vi "WS1021 GUI.vi"() -> ()   [LabVIEW 2020, in "WS1021.lvclass"]
uses:
  WS1021.lvclass
  C:/Sandbox/Git_Sandbox/WiSpry Test Framework source code (LV20)/WiSpry Test Framework/Devices/PIC-device/PIC-Device.lvclass
  C:/Sandbox/Git_Sandbox/WiSpry Test Framework source code (LV20)/WiSpry Test Framework/Devices/Toggle 8/Toggle 8.lvclass
  C:/Sandbox/Git_Sandbox/WiSpry Test Framework source code (LV20)/WiSpry Test Framework/Devices/Device.lvclass
  Controls/Register to Write.ctl
  PIC-device/PIC-Device.lvclass/PIC-Device.ctl
  Private/Get register for reading - array.vi
  PIC-device/PIC-Device.lvclass
  Toggle 8.lvclass
panel:
  in  "Init part":bool
  out "Y":i32
  out "X":i32
  in  "All reg 2 & 3":bool
  in  "Beam control mode":enum32{"OTP calibration", "Direct control"}(radio)
  in  "All reg3":bool
  in  "All reg2":bool
  in  "Reg3 beams":string="TB1 \n1/4pF\n\nTB2 \n1/4pF\n\nTB3\n1/4pF\n\nTB4\n1/4pF\n\nTB5\n1/4pF\n\nFB3\n1/8pF\n\nFB1 \n1/32pF"
  in  "Reg2 beams":string="TB6 \n1/4pF\n\nTB7 \n1/4pF\n\nTB8 \n1/4pF\n\nTB9 \n1/4pF\n\nTB10 \n1/4pF\n\nTB11 \n1/4pF\n\nFB2 \n1/16pF"
  in  "Reg3":bool[](array[boolean])=[FALSE, FALSE, FALSE, FALSE, FALSE, FALSE, FALSE]
  in  "Reg2":bool[](array[boolean])=[FALSE, FALSE, FALSE, FALSE, FALSE, FALSE, FALSE]
  in  "Stop Button":bool
  out "Boolean":bool
  out "Cycle":i32=1
  in  "Cycles":i32=1
  in  "USID":bool=TRUE
  out "Connected":bool
  out "SN#":string
  out "Product ID":string
  out "Manufacturer ID":string
  in  "Read info [F5]":bool
  in  "Close connection":bool
  in  "Toggle beams":bool
  in  "OTP values to read":string="0:127/1"
  in  "Read OTP":bool
  in  "Toggle Cmin/Cmax":bool
  in  "Init":bool
  out "Error Out":errorcluster
  in  "Error In":errorcluster
  in  "Write":bool
  in  "Exit":bool
  in  "Read":bool
  in  "Read reg":string="076000"
  in  "Write reg":string="074220"
  out "Cmd Send out":string
  in  "VISA resource name":refnum<visa-resource-name>
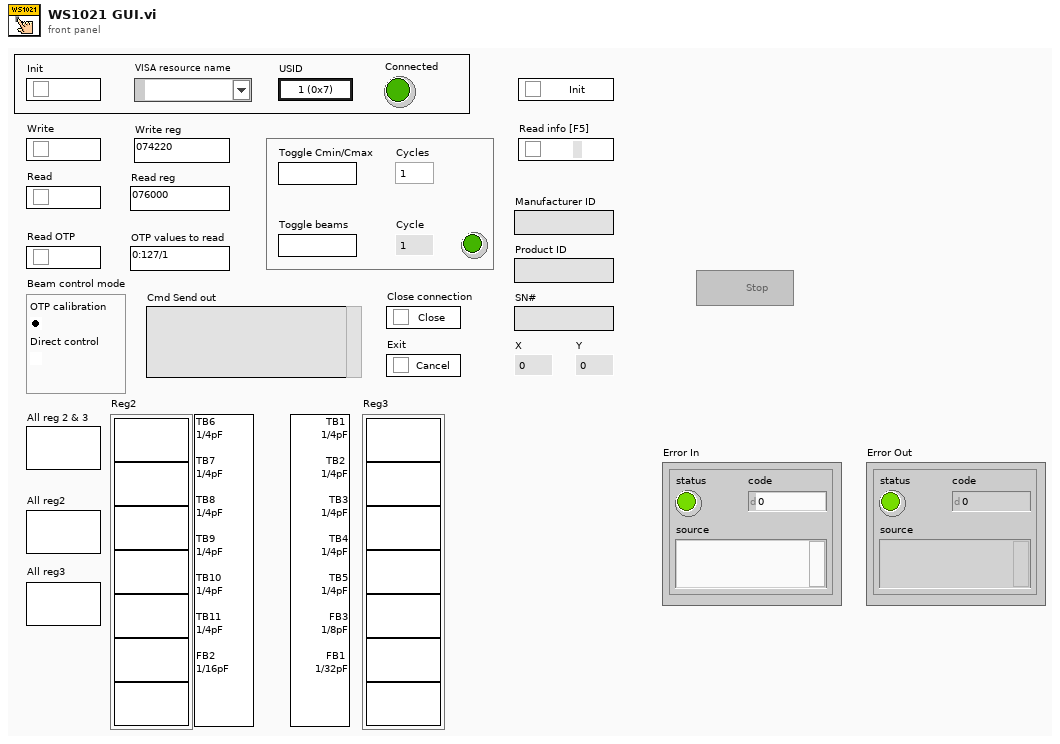
[diagram p1: front panel]
types:
  T1 = typedef "PIC-Device.lvclass/Register to Write.ctl" = cluster{"Register":u32, "Value":u32, "Dev Address":u32, "Physical Adress":u32}
  T2 = enum8{"Enabled", "Disabled", "Disabled and Grayed Out"}
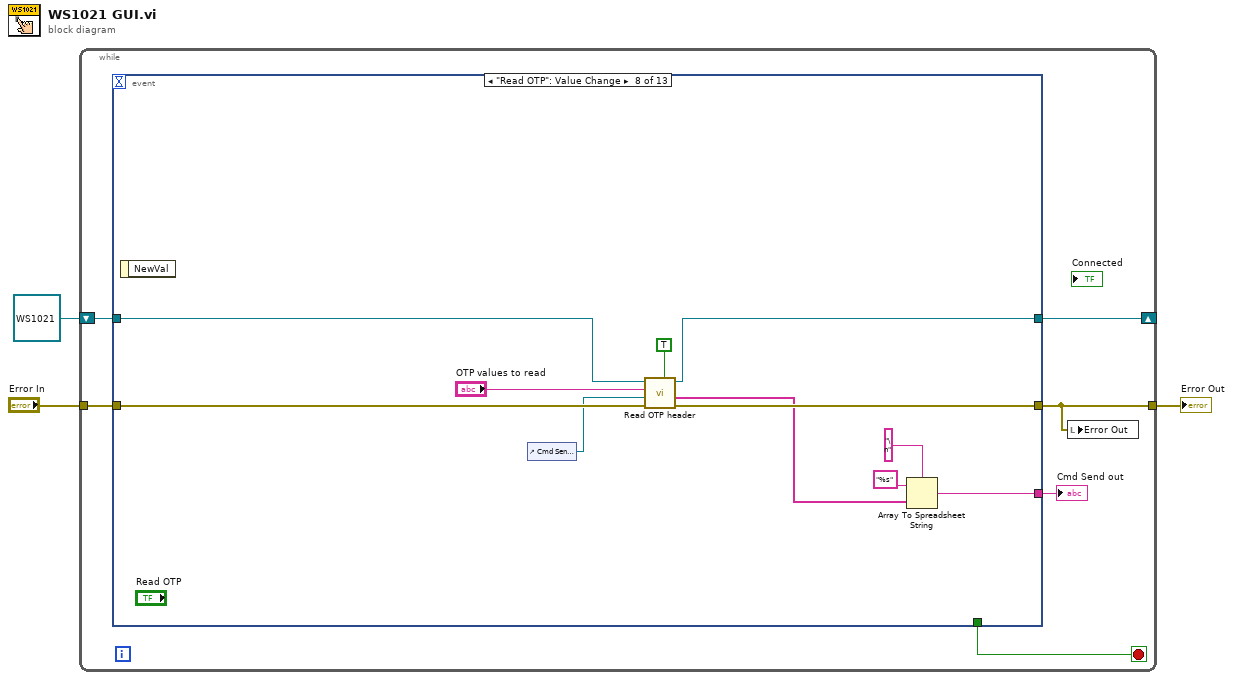
[diagram p0: block diagram]
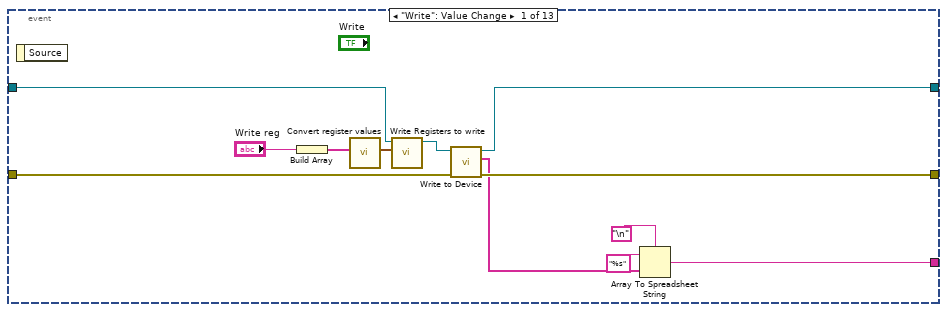
[diagram p2: hidden frame]
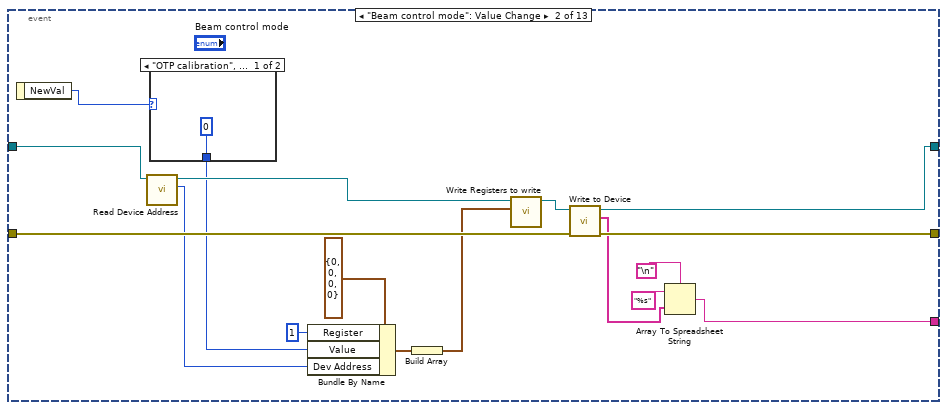
[diagram p3: hidden frame]
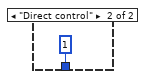
[diagram p4: hidden frame]
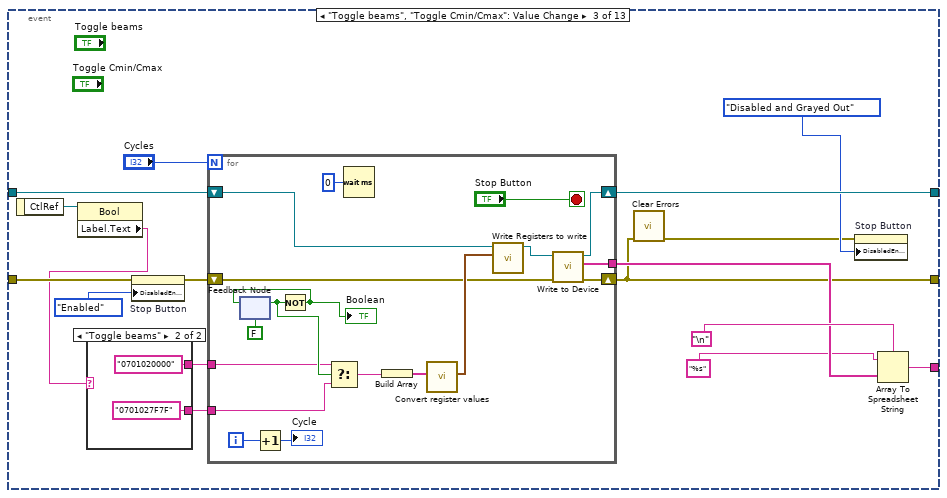
[diagram p5: hidden frame]
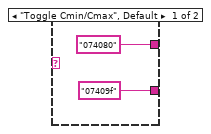
[diagram p6: hidden frame]
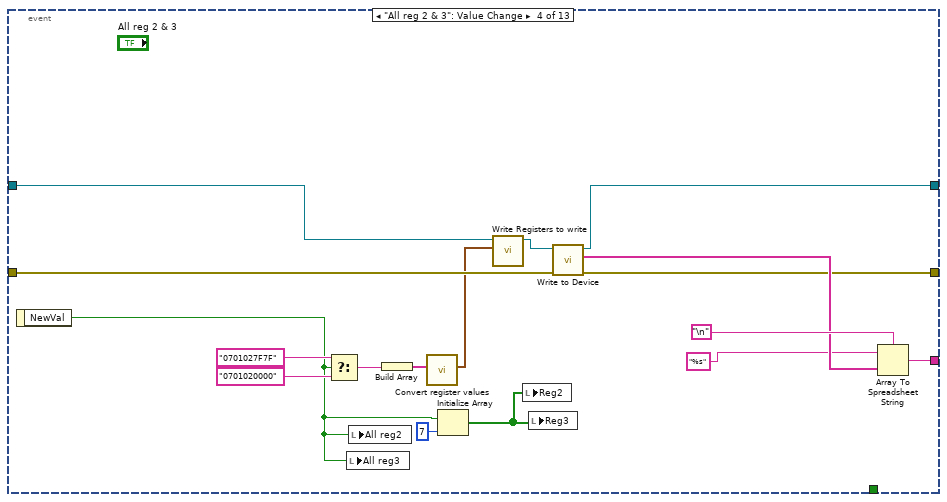
[diagram p7: hidden frame]
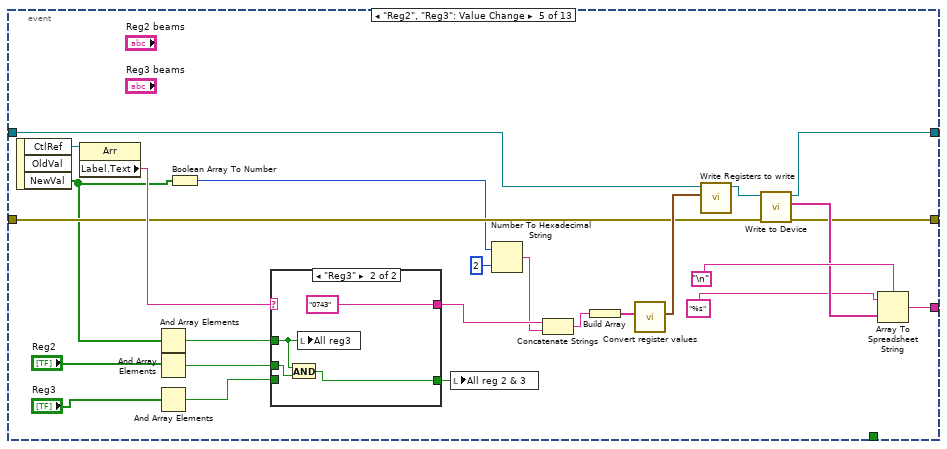
[diagram p8: hidden frame]
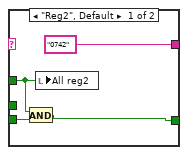
[diagram p9: hidden frame]
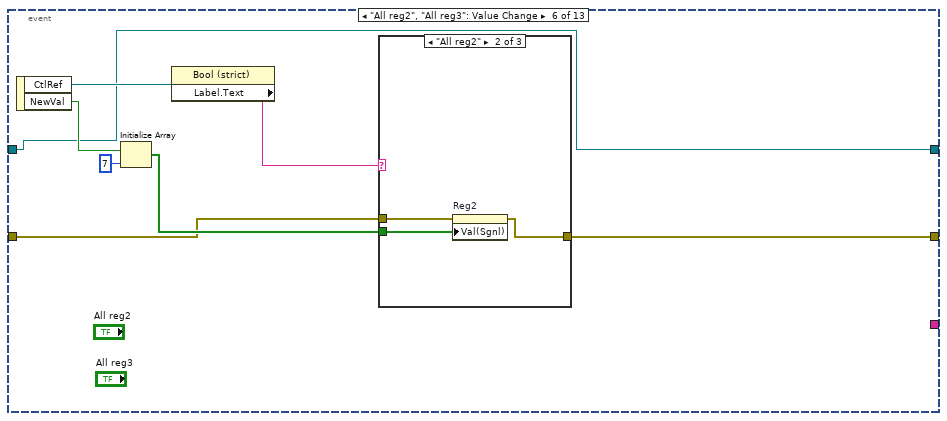
[diagram p10: hidden frame]
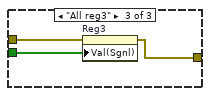
[diagram p12: hidden frame]
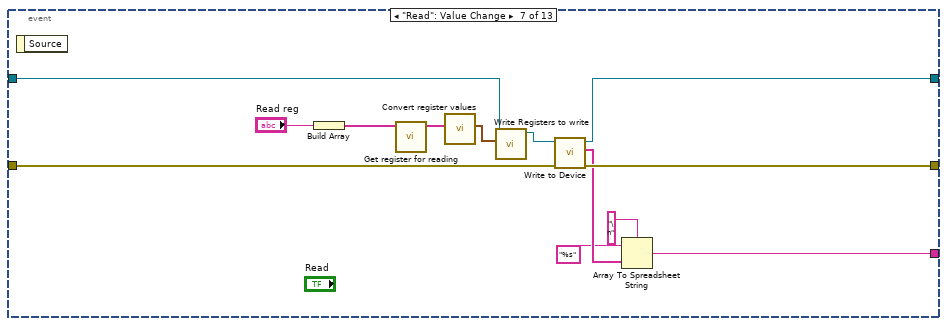
[diagram p13: hidden frame]
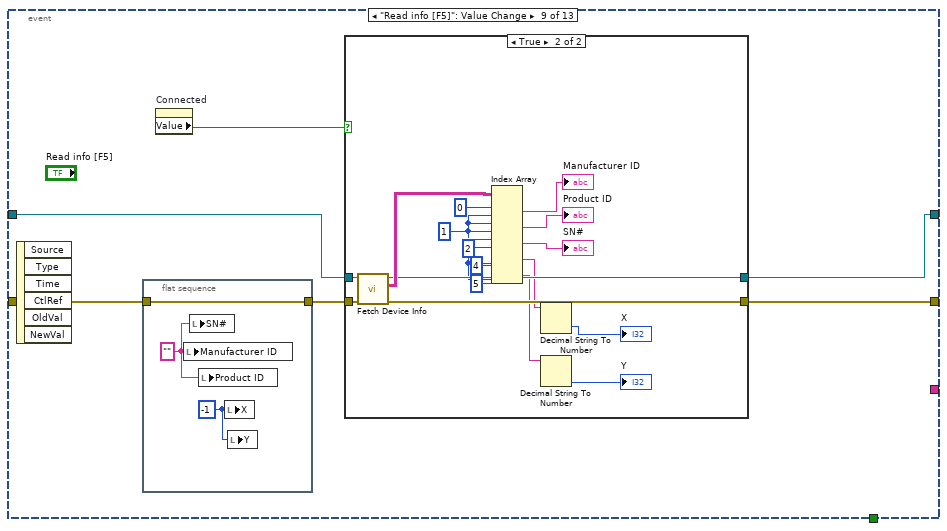
[diagram p14: hidden frame]
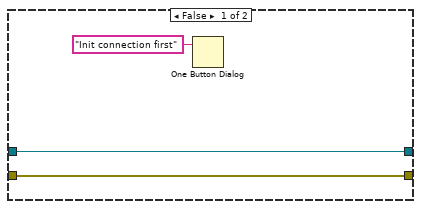
[diagram p15: hidden frame]
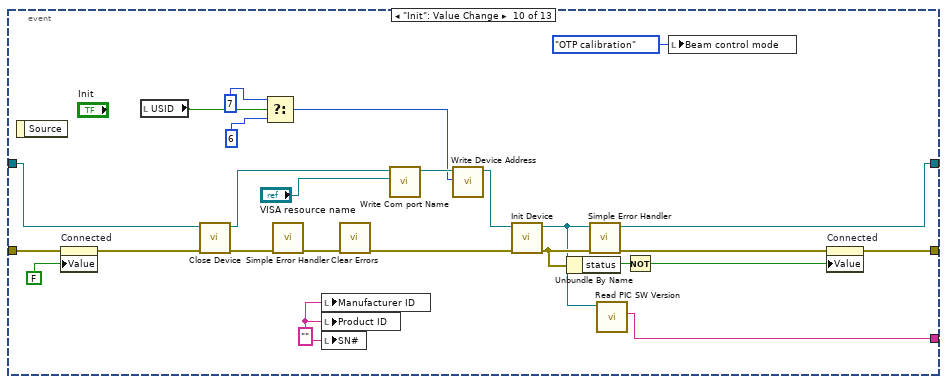
[diagram p16: hidden frame]
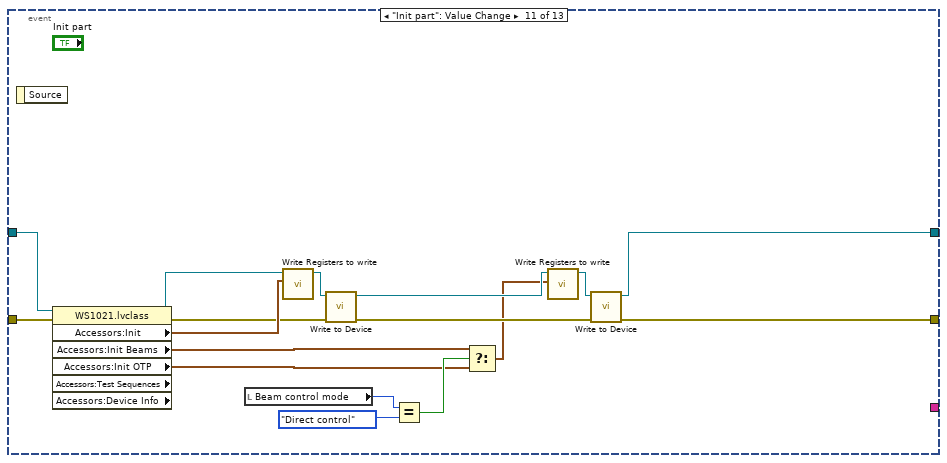
[diagram p17: hidden frame]
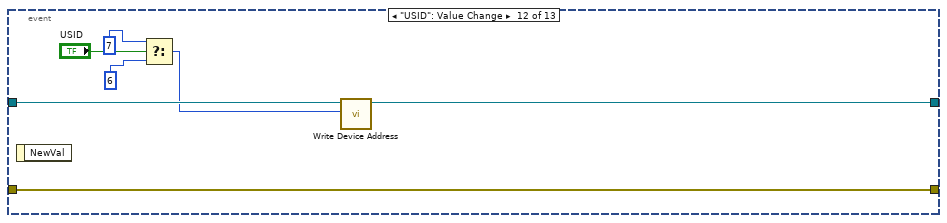
[diagram p18: hidden frame]
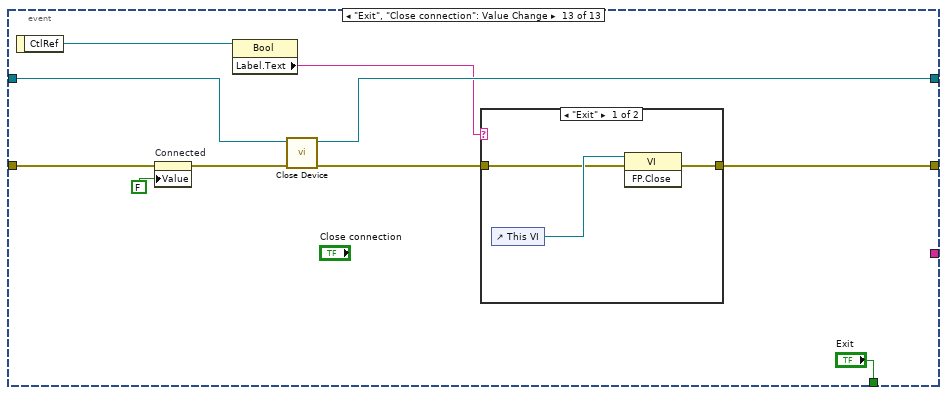
[diagram p19: hidden frame]
diagram:
  n1 = while {
    tunnel: "Error In" -> [w7]
    tunnel: [w6] -> w2
    shift-right: [w4] -> _
    shift-left: refnum<class "WS1021.lvclass"> refnum ("WS1021.lvclass") -> [w5]
    stop <- w8 stop-if-true
    n2 = event shown="[7] \"Read OTP\": Value Change" {
      selector: _ -> [_ _ _ _ _ _ _ _ _ _ _ _ _]
      dyn-events: _ -> [_ _ _ _ _ _ _ _ _ _ _ _ _]
      timeout: _ -> [_ _ _ _ _ _ _ _ _ _ _ _ _]
      tunnel: w7 -> [w18 w36 w53 w94 w109 w131 w154 w168 w174 w217 w237 w243 w254]
      tunnel: [w21 w35 w46 w89 w115 w132 w155 w167 w173 w220 w225 w243 w248] -> w6
      tunnel: [w11 w22 w47 w90 w116 _ w148 w163 _ w199 _ _ _] -> w9
      tunnel: [_ _ _ _ _ _ _ _ _ _ _ _ "Exit"] -> w8
      tunnel: w5 -> [w10 w34 w56 w95 w120 w130 w146 w161 w171 w211 w238 w245 w251]
      tunnel: [w17 w26 w57 w96 w121 w130 w145 w160 w170 w200 w224 w244 w250] -> w4
      event "Write": Value Change {
        n3 = event-data() -> ()  [unwired: 1 in, 1 out]
        n4 = Build Array("Write reg") -> (w15:string[])
        n5 = call "Convert register values.vi"("Register strings"=w15) -> ("Register clusters out"=w20:T1[])  [unwired: 9 in, 1 out]
        n6 = call-dynamic "Write Registers to write.vi"("Registers to write"=w20, "Device in"=w10) -> ("Device out"=w19:refnum<class "WS1021.lvclass">)  [unwired: 9 in]
        n7 = call-dynamic "Write to Device.vi"("error in (no error)"=w18, "Device in"=w19) -> ("error out"=w21:errorcluster, "Return"=w12:string[], "Device out"=w17:refnum<class "WS1021.lvclass">)  [unwired: 7 in]
        n8 = Array To Spreadsheet String(delimiter (Tab)="\n", array=w12, 3:"%s" ("format string")) -> (spreadsheet string=w11:string)
      }
      event "Beam control mode": Value Change {
        n9 = event-data() -> ("NewVal"=w38:enum32{"OTP calibration", "Direct control"})  [unwired: 1 in]
        n10 = call-dynamic "Read Device Address.vi"("PIC-Device in"=w34) -> ("Device Address"=w32:u8, "PIC-Device out"=w31:refnum<class "WS1021.lvclass">)  [unwired: 9 in]
        n11 = case shown="\"OTP calibration\", Default" w38 {
          tunnel: [u32 0 ("Value") u32 1 ("Value")] -> w29
          frame "OTP calibration", Default {
          }
          frame "Direct control" {
          }
        }
        n12 = Bundle By Name(cluster=T1 {"Register"=0, "Value"=0, "Dev Address"=0, "Physical Adress"=0} ("Register to Write"), "Register"=u32 1, "Value"=w29, "Dev Address"=w32) -> (w28:T1)
        n13 = Build Array(w28) -> (w27:T1[])
        n14 = call-dynamic "Write Registers to write.vi"("Registers to write"=w27, "Device in"=w31) -> ("Device out"=w37:refnum<class "WS1021.lvclass">)  [unwired: 9 in]
        n15 = call-dynamic "Write to Device.vi"("error in (no error)"=w36, "Device in"=w37) -> ("error out"=w35:errorcluster, "Return"=w23:string[], "Device out"=w26:refnum<class "WS1021.lvclass">)  [unwired: 7 in]
        n16 = Array To Spreadsheet String(delimiter (Tab)="\n", array=w23, 3:"%s" ("format string")) -> (spreadsheet string=w22:string)
      }
      event "Toggle beams", "Toggle Cmin/Cmax": Value Change {
        n17 = event-data() -> ("CtlRef"=w44:refnum<vi>)  [unwired: 1 in]
        n18 = property class="Bool"(reference=w44) -> ("Label.Text"=w43:string)  [unwired: 1 in, 2 out]
        n19 = case shown="\"Toggle beams\"" w43 {
          tunnel: ["074080" ("Write reg 2") "0701020000" ("Write reg 2")] -> w42
          tunnel: ["07409f" ("Write reg 2") "0701027F7F" ("Write reg 2")] -> w41
          frame "Toggle Cmin/Cmax", Default {
          }
          frame "Toggle beams" {
          }
        }
        n20 = property on="Stop Button" class="Bool"(error in=w53, "DisabledEnum"=T2."Enabled" ("Disabled")) -> (error out=w52:errorcluster)  [unwired: 1 in, 1 out]
        n21 = for {
          N: "Cycles" -> [_]
          shift-right: [w75] -> w46
          shift-left: w52 -> [w73]
          shift-right: [w74] -> w57
          shift-left: w56 -> [w71]
          tunnel: [w67] -> w49
          tunnel: w42 -> [w66]
          tunnel: w41 -> [w65]
          i -> [w70]
          stop <- "Stop Button" stop-if-true
          n22 = feedback #1(FALSE) -> (w68:bool)
          n23 = Increment(x=w70) -> (x+1=→"Cycle":i32)
          n24 = Not(x=w68) -> (.not. x?=w62:bool)
          "Boolean" <- w62
          n25 = feedback-in #1(w62) -> ()
          n26 = Select(t=w66, s=w68, f=w65) -> (s? t:f=w72:string)
          n27 = Wait (ms)(milliseconds to wait=u32 0) -> ()  [unwired: 1 out]
          n28 = Build Array(w72) -> (w76:string[])
          n29 = call "Convert register values.vi"("Register strings"=w76) -> ("Register clusters out"=w77:T1[])  [unwired: 9 in, 1 out]
          n30 = call-dynamic "Write Registers to write.vi"("Registers to write"=w77, "Device in"=w71) -> ("Device out"=w78:refnum<class "WS1021.lvclass">)  [unwired: 9 in]
          n31 = call-dynamic "Write to Device.vi"("error in (no error)"=w73, "Device in"=w78) -> ("error out"=w75:errorcluster, "Return"=w67:string[], "Device out"=w74:refnum<class "WS1021.lvclass">)  [unwired: 7 in]
        }
        n32 = call <vilib>:"Clear Errors.vi"("error in (no error)"=w46) -> ("error out"=w45:errorcluster)  [unwired: 5 in, 1 out]
        n33 = property on="Stop Button" class="Bool"(error in=w45, "DisabledEnum"=T2."Disabled and Grayed Out" ("Disabled")) -> ()  [unwired: 1 in, 2 out]
        n34 = Array To Spreadsheet String(delimiter (Tab)="\n", array=w49, 3:"%s" ("format string")) -> (spreadsheet string=w47:string)
      }
      event "All reg 2 & 3": Value Change {
        n35 = event-data() -> ("NewVal"=w80:bool)  [unwired: 1 in]
        n36 = Select(t="0701027F7F" ("Write reg 2"), s=w80, f="0701020000" ("Write reg 2")) -> (s? t:f=w83:string)
        n37 = local write "All reg3"(w80) -> ()
        n38 = local write "All reg2"(w80) -> ()
        n39 = Build Array(w83) -> (w84:string[])
        n40 = call "Convert register values.vi"("Register strings"=w84) -> ("Register clusters out"=w85:T1[])  [unwired: 9 in, 1 out]
        n41 = Initialize Array(w80, 7 ("dimension size")) -> (w81:bool[])
        n42 = call-dynamic "Write Registers to write.vi"("Registers to write"=w85, "Device in"=w95) -> ("Device out"=w86:refnum<class "WS1021.lvclass">)  [unwired: 9 in]
        n43 = local write "Reg2"(w81) -> ()
        n44 = local write "Reg3"(w81) -> ()
        n45 = call-dynamic "Write to Device.vi"("error in (no error)"=w94, "Device in"=w86) -> ("error out"=w89:errorcluster, "Return"=w92:string[], "Device out"=w96:refnum<class "WS1021.lvclass">)  [unwired: 7 in]
        n46 = Array To Spreadsheet String(delimiter (Tab)="\n", array=w92, 3:"%s" ("format string")) -> (spreadsheet string=w90:string)
      }
      event "Reg2", "Reg3": Value Change {
        n47 = event-data() -> ("CtlRef"=w114:refnum<vi>, "NewVal"=w103:bool[])  [unwired: 1 in, 1 out]
        n48 = property class="Arr"(reference=w114) -> ("Label.Text"=w113:string)  [unwired: 1 in, 2 out]
        n49 = And Array Elements(Boolean array=w103) -> (logical AND=w102:bool)
        n50 = And Array Elements(Boolean array="Reg2") -> (logical AND=w98:bool)
        n51 = And Array Elements(Boolean array="Reg3") -> (logical AND=w99:bool)
        n52 = Boolean Array To Number(Boolean array=w103) -> (number=w107:u32)
        n53 = case shown="\"Reg3\"" w113 {
          tunnel: ["0742" ("Write reg 2") "0743" ("Write reg 2")] -> w106
          tunnel: w102 -> [w124 w128]
          tunnel: w99 -> [w123 _]
          tunnel: w98 -> [_ w127]
          tunnel: [w122 w126] -> w97
          frame "Reg2", Default {
            n54 = And(x=w124, y=w123) -> (x .and. y?=w122:bool)
            n55 = local write "All reg2"(w124) -> ()
          }
          frame "Reg3" {
            n56 = And(x=w128, y=w127) -> (x .and. y?=w126:bool)
            n57 = local write "All reg3"(w128) -> ()
          }
        }
        n58 = local write "All reg 2 & 3"(w97) -> ()
        n59 = Number To Hexadecimal String(1:i16 2 ("width (-)"), 2:w107) -> (0:w105:string)
        n60 = Concatenate Strings(w106, w105) -> (w104:string)
        n61 = Build Array(w104) -> (w110:string[])
        n62 = call "Convert register values.vi"("Register strings"=w110) -> ("Register clusters out"=w111:T1[])  [unwired: 9 in, 1 out]
        n63 = call-dynamic "Write Registers to write.vi"("Registers to write"=w111, "Device in"=w120) -> ("Device out"=w112:refnum<class "WS1021.lvclass">)  [unwired: 9 in]
        n64 = call-dynamic "Write to Device.vi"("error in (no error)"=w109, "Device in"=w112) -> ("error out"=w115:errorcluster, "Return"=w118:string[], "Device out"=w121:refnum<class "WS1021.lvclass">)  [unwired: 7 in]
        n65 = Array To Spreadsheet String(delimiter (Tab)="\n", array=w118, 3:"%s" ("format string")) -> (spreadsheet string=w116:string)
      }
      event "All reg2", "All reg3": Value Change {
        n66 = event-data() -> ("CtlRef"=w137:refnum<vi>, "NewVal"=w135:bool)  [unwired: 1 in]
        n67 = Initialize Array(w135, 7 ("dimension size")) -> (w133:bool[])
        n68 = property class="Bool (strict)"(reference=w137) -> ("Label.Text"=w136:string)  [unwired: 1 in, 2 out]
        n69 = case shown="\"All reg2\"" w136 {
          tunnel: w133 -> [_ w141 w144]
          tunnel: [w138 w139 w143] -> w132
          tunnel: w131 -> [w138 w140 w142]
          frame Default {
          }
          frame "All reg2" {
            n70 = property on="Reg2" class="Arr"(error in=w140, "Val(Sgnl)"=w141) -> (error out=w139:errorcluster)  [unwired: 1 in, 1 out]
          }
          frame "All reg3" {
            n71 = property on="Reg3" class="Arr"(error in=w142, "Val(Sgnl)"=w144) -> (error out=w143:errorcluster)  [unwired: 1 in, 1 out]
          }
        }
      }
      event "Read": Value Change {
        n72 = event-data() -> ()  [unwired: 1 in, 1 out]
        n73 = Build Array("Read reg") -> (w151:string[])
        n74 = call-poly "Get register for reading.vi"("Reg array in"=w151) -> ("Reg array out"=w153:string[])  [unwired: 10 in]
        n75 = call "Convert register values.vi"("Register strings"=w153) -> ("Register clusters out"=w157:T1[])  [unwired: 9 in, 1 out]
        n76 = call-dynamic "Write Registers to write.vi"("Registers to write"=w157, "Device in"=w146) -> ("Device out"=w156:refnum<class "WS1021.lvclass">)  [unwired: 9 in]
        n77 = call-dynamic "Write to Device.vi"("error in (no error)"=w154, "Device in"=w156) -> ("error out"=w155:errorcluster, "Return"=w149:string[], "Device out"=w145:refnum<class "WS1021.lvclass">)  [unwired: 7 in]
        n78 = Array To Spreadsheet String(delimiter (Tab)="\n", array=w149, 3:"%s" ("format string")) -> (spreadsheet string=w148:string)
      }
      event "Read OTP": Value Change {
        n79 = event-data() -> ()  [unwired: 1 in, 1 out]
        n80 = control-ref of="Cmd Send out"() -> (w159:refnum<vi>)
        n81 = call-dynamic "Read OTP header.vi"("Write to file"=TRUE, "error in (no error)"=w168, "reference"=w159, "OTP values to read"="OTP values to read", "PIC-Device in"=w161) -> ("error out"=w167:errorcluster, "Array"=w166:string[], "PIC-Device out"=w160:refnum<class "WS1021.lvclass">)  [unwired: 4 in]
        n82 = Array To Spreadsheet String(delimiter (Tab)="\n", array=w166, 3:"%s" ("format string")) -> (spreadsheet string=w163:string)
      }
      event "Read info [F5]": Value Change {
        n83 = event-data() -> ()  [unwired: 1 in, 6 out]
        n84 = flat-sequence {
          tunnel: w174 -> [w196]
          tunnel: [w196] -> w172
          frame #0 {
            w195 = -1 ("X")
            w197 = "" ("Manufacturer ID")
            n85 = local write "Manufacturer ID"(w197) -> ()
            n86 = local write "SN#"(w197) -> ()
            n87 = local write "Product ID"(w197) -> ()
            n88 = local write "X"(w195) -> ()
            n89 = local write "Y"(w195) -> ()
          }
        }
        n90 = property on="Connected" class="Bool (strict)"() -> ("Value"=w169:bool)  [unwired: 2 in, 2 out]
        n91 = case shown="True" w169 {
          tunnel: [w176 w190] -> w173
          tunnel: w172 -> [w176 w189]
          tunnel: w171 -> [w175 w188]
          tunnel: [w175 w187] -> w170
          frame False {
            n92 = One Button Dialog(message="Init connection first") -> ()  [unwired: 1 in, 1 out]
          }
          frame True {
            w184 = 1 ("disabled index (col)")
            n93 = call-dynamic "Fetch Device Info.vi"("error in (no error)"=w189, "Toggle 8 in"=w188) -> ("error out"=w190:errorcluster, "Device Info"=w194:string[][], "Toggle 8 out"=w187:refnum<class "WS1021.lvclass">)  [unwired: 7 in]
            n94 = Index Array(array=w194, index (row) #1=0 ("disabled index (row)"), index (col) #1=w184, index (row) #2=w184, index (col) #2=w184, index (row) #3=2 ("disabled index (row)"), index (col) #3=w184, index (row) #4=4 ("disabled index (row)"), index (col) #4=w184, index (row) #5=5 ("disabled index (row)"), index (col) #5=w184) -> (element #1=→"Manufacturer ID":string, element #2=→"Product ID":string, element #3=→"SN#":string, element #4=w181:string, element #5=w180:string)
            n95 = Decimal String To Number(string=w181) -> (number=→"X":i32)  [unwired: 2 in, 1 out]
            n96 = Decimal String To Number(string=w180) -> (number=→"Y":i32)  [unwired: 2 in, 1 out]
          }
        }
      }
      event "Init": Value Change {
        w201 = "" ("Product ID")
        n97 = event-data() -> ()  [unwired: 1 in, 1 out]
        n98 = property on="Connected" class="Bool (strict)"(error in=w217, "Value"=FALSE ("Connected")) -> (error out=w213:errorcluster)  [unwired: 1 in, 1 out]
        n99 = local read "USID"() -> (w205:bool)
        n100 = call-dynamic "Close Device.vi"("error in (no error)"=w213, "Device in"=w211) -> ("error out"=w212:errorcluster, "Device out"=w210:refnum<class "WS1021.lvclass">)  [unwired: 8 in]
        n101 = Select(t=u8 7 ("Device Address"), s=w205, f=u8 6 ("Device Address")) -> (s? t:f=w204:u8)
        n102 = call <vilib>:"Simple Error Handler.vi"("error in (no error)"=w212) -> ("error out"=w221:errorcluster)  [unwired: 4 in, 4 out]
        n103 = local write "Manufacturer ID"(w201) -> ()
        n104 = local write "Product ID"(w201) -> ()
        n105 = local write "SN#"(w201) -> ()
        n106 = call <vilib>:"Clear Errors.vi"("error in (no error)"=w221) -> ("error out"=w214:errorcluster)  [unwired: 5 in, 1 out]
        n107 = call-dynamic "Write Com port Name.vi"("Com port Name"="VISA resource name", "Device in"=w210) -> ("Device out"=w209:refnum<class "WS1021.lvclass">)  [unwired: 9 in]
        n108 = call-dynamic "Write Device Address.vi"("Device Address"=w204, "PIC-Device in"=w209) -> ("PIC-Device out"=w208:refnum<class "WS1021.lvclass">)  [unwired: 9 in]
        n109 = call-dynamic "Init Device.vi"("error in (no error)"=w214, "Toggle 8 in"=w208) -> ("error out"=w203:errorcluster, "Toggle 8 out"=w200:refnum<class "WS1021.lvclass">)  [unwired: 8 in]
        n110 = Unbundle By Name(w203) -> ("status"=w219:bool)
        n111 = call <vilib>:"Simple Error Handler.vi"("error in (no error)"=w203) -> ("error out"=w202:errorcluster)  [unwired: 4 in, 4 out]
        n112 = call "Read PIC SW Version.vi"("Device in"=w200) -> ("PIC SW Version"=w199:string)  [unwired: 9 in, 1 out]
        n113 = Not(x=w219) -> (.not. x?=w218:bool)
        n114 = local write "Beam control mode"(enum32{"OTP calibration", "Direct control"}."OTP calibration" ("Beam control mode")) -> ()
        n115 = property on="Connected" class="Bool (strict)"(error in=w202, "Value"=w218) -> (error out=w220:errorcluster)  [unwired: 1 in, 1 out]
      }
      event "Init part": Value Change {
        n116 = event-data() -> ()  [unwired: 1 in, 1 out]
        n117 = property class="WS1021.lvclass" props=["Accessors:Init", "Accessors:Init Beams", "Accessors:Init OTP", "Accessors:Test Sequences", "Accessors:Device Info"](reference=w238, error in=w237) -> (reference out=w232:refnum<class "WS1021.lvclass">, error out=w233:errorcluster, "Accessors:Init"=w234:T1[], "Accessors:Init Beams"=w230:T1[], "Accessors:Init OTP"=w226:T1[])  [unwired: 2 out]
        n118 = local read "Beam control mode"() -> (w228:enum32{"OTP calibration", "Direct control"})
        n119 = call-dynamic "Write Registers to write.vi"("Registers to write"=w234, "Device in"=w232) -> ("Device out"=w236:refnum<class "WS1021.lvclass">)  [unwired: 9 in]
        n120 = call-dynamic "Write to Device.vi"("error in (no error)"=w233, "Device in"=w236) -> ("error out"=w231:errorcluster, "Device out"=w223:refnum<class "WS1021.lvclass">)  [unwired: 7 in, 1 out]
        n121 = Equal?(x=w228, y=enum32{"OTP calibration", "Direct control"}."Direct control" ("Beam control mode")) -> (x = y?=w227:bool)
        n122 = Select(t=w230, s=w227, f=w226) -> (s? t:f=w222:T1[])
        n123 = call-dynamic "Write Registers to write.vi"("Registers to write"=w222, "Device in"=w223) -> ("Device out"=w235:refnum<class "WS1021.lvclass">)  [unwired: 9 in]
        n124 = call-dynamic "Write to Device.vi"("error in (no error)"=w231, "Device in"=w235) -> ("error out"=w225:errorcluster, "Device out"=w224:refnum<class "WS1021.lvclass">)  [unwired: 7 in, 1 out]
      }
      event "USID": Value Change {
        n125 = event-data() -> ()  [unwired: 1 in, 1 out]
        n126 = Select(t=u8 7 ("Device Address"), s="USID", f=u8 6 ("Device Address")) -> (s? t:f=w239:u8)
        n127 = call-dynamic "Write Device Address.vi"("Device Address"=w239, "PIC-Device in"=w245) -> ("PIC-Device out"=w244:refnum<class "WS1021.lvclass">)  [unwired: 9 in]
      }
      event "Exit", "Close connection": Value Change {
        n128 = event-data() -> ("CtlRef"=w247:refnum<vi>)  [unwired: 1 in]
        n129 = property on="Connected" class="Bool (strict)"(error in=w254, "Value"=FALSE ("Connected")) -> (error out=w252:errorcluster)  [unwired: 1 in, 1 out]
        n130 = property class="Bool"(reference=w247) -> ("Label.Text"=w246:string)  [unwired: 1 in, 2 out]
        n131 = call-dynamic "Close Device.vi"("error in (no error)"=w252, "Device in"=w251) -> ("error out"=w249:errorcluster, "Device out"=w250:refnum<class "WS1021.lvclass">)  [unwired: 8 in]
        n132 = case shown="\"Exit\"" w246 {
          tunnel: w249 -> [w257 w259]
          tunnel: [w256 w259] -> w248
          frame "Exit" {
            n133 = control-ref of="This VI"() -> (w258:refnum<vi>)
            n134 = invoke class="VI" method="FP.Close"(reference=w258, error in=w257) -> (error out=w256:errorcluster)  [unwired: 1 in, 2 out]
          }
          frame Default {
          }
        }
      }
    }
    "Cmd Send out" <- w9
    n135 = local write "Error Out"(w6) -> ()
  }
  "Error Out" <- w2
